vi "RPM_Claim.vi"() -> ()   [LabVIEW 2020]
uses:
  <vilib>/Instr/_visa.llb/VISA Configure Serial Port (Instr).vi
panel:
  out "number":dbl
  out "after substring":string
  out "read buffer":string
  out "RPM":dbl(knob) scale=0.0..150.0
  in  "stop":bool
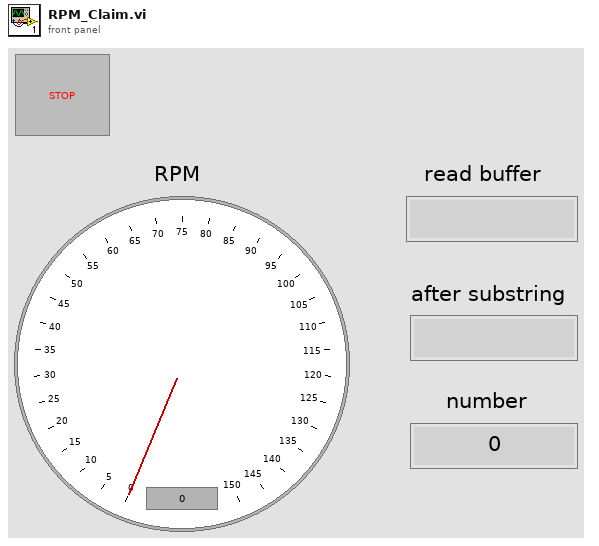
[diagram p1: front panel]
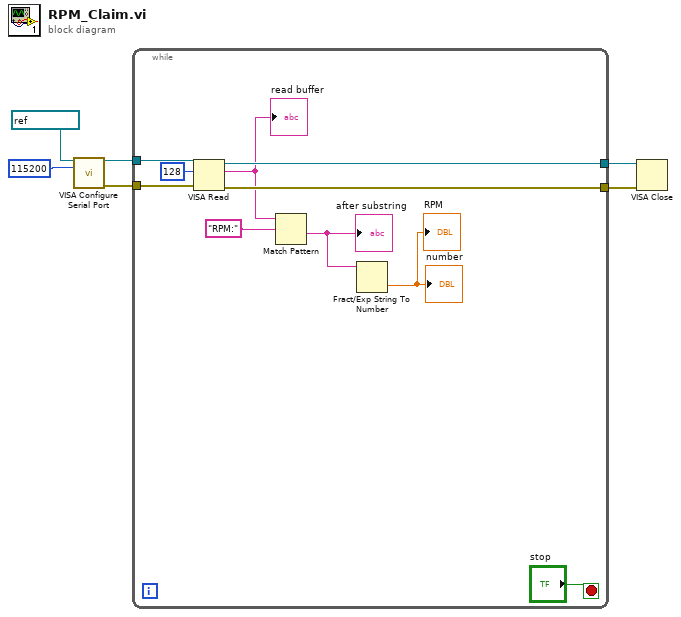
[diagram p0: block diagram]
diagram:
  n1 = call-poly "VISA Configure Serial Port"("VISA resource name"=refnum<visa-resource-name> "COM12", "baud rate (9600)"=u32 115200) -> ("VISA resource name out"=w5:refnum<visa-resource-name>, "error out"=w4:errorcluster)  [unwired: 12 in]
  n2 = while {
    tunnel: w5 -> [w15]
    tunnel: w4 -> [w14]
    tunnel: [w13] -> w3
    tunnel: [w12] -> w2
    stop <- "stop" stop-if-true
    n3 = VISA Read(VISA resource name=w15, byte count=u32 128, error in (no error)=w14) -> (VISA resource name out=w13:refnum<visa-resource-name>, read buffer=w10:string, error out=w12:errorcluster)  [unwired: 1 out]
    "read buffer" <- w10
    n4 = Match Pattern(string=w10, regular expression="RPM:") -> (after substring=w8:string)  [unwired: 1 in, 3 out]
    "after substring" <- w8
    n5 = Fract/Exp String To Number(string=w8) -> (number=→"RPM" →"number":dbl)  [unwired: 3 in, 1 out]
  }
  n6 = VISA Close(VISA resource name=w3, error in (no error)=w2) -> ()  [unwired: 1 out]
